vi "importAcq.vi"(8 "error in (no error)":errorcluster, 11 "Acquisition in":refnum<class "Acquisition.lvclass">) -> (0 "error out":errorcluster, 2 "# elements in queue":i32, 3 "Acquisition out":refnum<class "Acquisition.lvclass">)   [LabVIEW 2014, in "Acquisition.lvclass"]
uses:
  Acquisition.lvclass
  Acquisition.lvclass/Acquisition.ctl
  Database/Database.lvclass
panel:
  in  "Tuple":T1={"mouse_id"=1217.0, "session_timestamp"="", "timestamp"=0.0, "stimulus"="", "trial"=0}
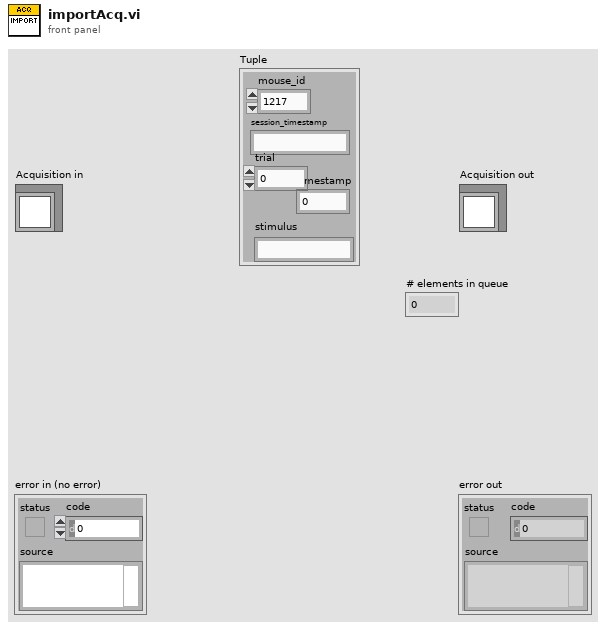
[diagram p1: front panel]
types:
  T1 = cluster{"mouse_id":dbl, "session_timestamp":string, "timestamp":dbl, "stimulus":string, "trial":u16}
  T2 = cluster{"timestamp":dbl, "stimulus":string, "trial":dbl}
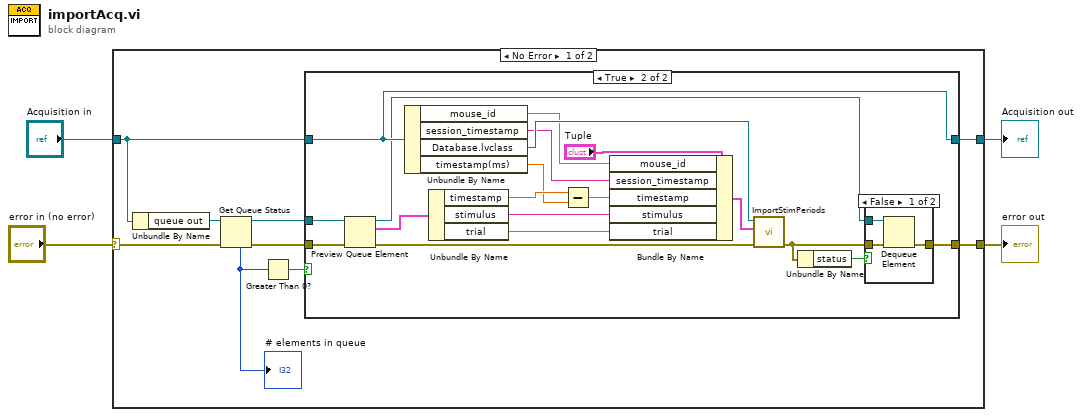
[diagram p0: block diagram]
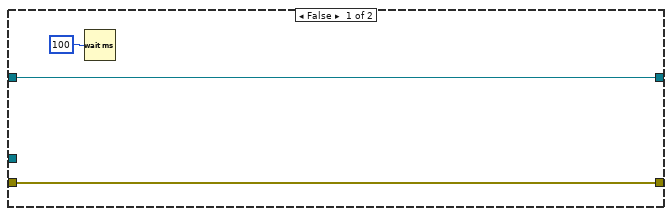
[diagram p2: hidden frame]
diagram:
  n1 = case shown="No Error" "error in (no error)" {
    selector: "error in (no error)" -> [w8 w41]
    tunnel: [w13 w41] -> w3
    tunnel: [w12 w40] -> w1
    tunnel: "Acquisition in" -> [w11 w40]
    frame No Error {
      n2 = Unbundle By Name(w11) -> ("queue out"=w10:refnum<queue>)
      n3 = Get Queue Status(queue=w10, error in (no error)=w8) -> (queue out=w9:refnum<queue>, error out=w7:errorcluster, # elements in queue=w6:i32)  [unwired: 1 in, 5 out]
      "# elements in queue" <- w6
      n4 = Greater Than 0?(x=w6) -> (x > 0?=w5:bool)
      n5 = case shown="True" w5 {
        tunnel: [w15 w32] -> w13
        tunnel: w9 -> [_ w35]
        tunnel: [w14 w25] -> w12
        tunnel: w11 -> [w14 w25]
        tunnel: w7 -> [w15 w34]
        frame False {
          n6 = Wait (ms)(milliseconds to wait=u32 100) -> ()  [unwired: 1 out]
        }
        frame True {
          n7 = Preview Queue Element(queue=w35, error in (no error)=w34) -> (queue out=w24:refnum<queue>, element=w27:T2, error out=w23:errorcluster)  [unwired: 1 in, 1 out]
          n8 = Unbundle By Name(w25) -> ("mouse_id"=w29:dbl, "session_timestamp"=w28:string, "Database.lvclass"=w30:refnum<class "Database.lvclass">, "timestamp(ms)"=w18:dbl)
          n9 = Unbundle By Name(w27) -> ("timestamp"=w19:dbl, "stimulus"=w26:string, "trial"=w20:dbl)
          n10 = Subtract(x=w19, y=w18) -> (x-y=w17:dbl)
          n11 = Bundle By Name(cluster="Tuple", "mouse_id"=w29, "session_timestamp"=w28, "timestamp"=w17, "stimulus"=w26, "trial"=w20) -> (w22:T1)
          n12 = call-dynamic "ImportStimPeriods.vi"("error in (no error)"=w23, "Tuple"=w22, "Database in"=w30) -> ("error out"=w33:errorcluster)  [unwired: 7 in, 1 out]
          n13 = Unbundle By Name(w33) -> ("status"=w31:bool)
          n14 = case shown="False" w31 {
            tunnel: w33 -> [w38 w39]
            tunnel: [w37 w39] -> w32
            tunnel: w24 -> [w36 _]
            frame False {
              n15 = Dequeue Element(queue=w36, error in (no error)=w38) -> (error out=w37:errorcluster)  [unwired: 1 in, 3 out]
            }
            frame True {
            }
          }
        }
      }
    }
    frame Error {
    }
  }
  "error out" <- w3
  "Acquisition out" <- w1
